vi "欧姆龙PLC通讯Fans UDP-写PLC寄存器编码-16bit寄存器.vi"(10 "数据U16":u16[](array[numeric]), 11 "起始地址16":string) -> (3 "写入数据编码":string)   [LabVIEW 2014]
panel:
  out "16bit寄存器个数":string
  out "字符串":string
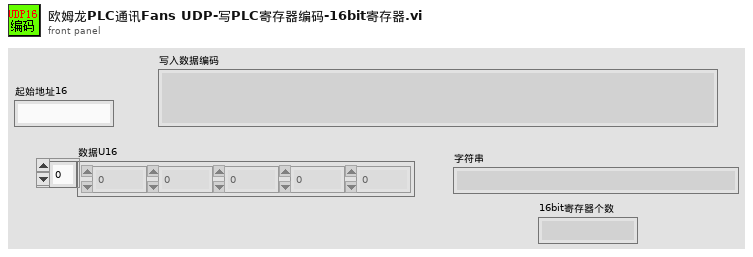
[diagram p1: front panel]
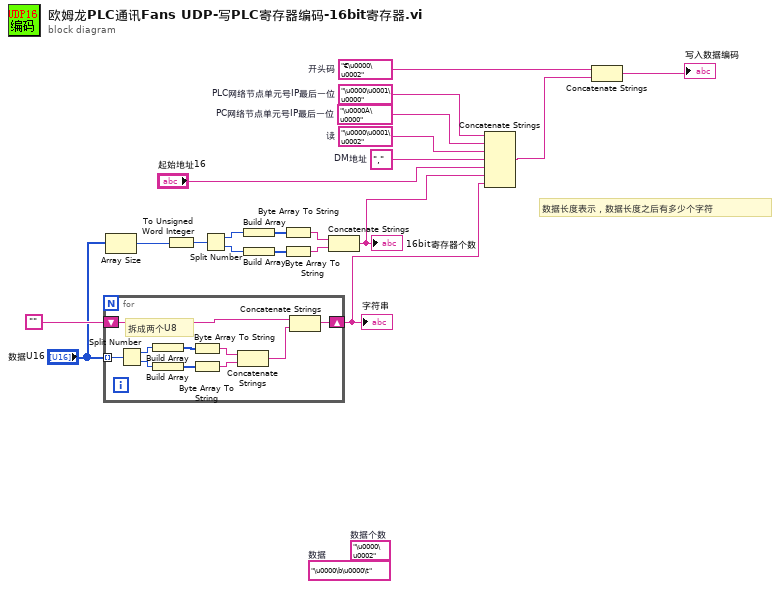
[diagram p0: block diagram]
diagram:
  w18 = "\u0000À\u0000"  # PC网络节点单元号IP最后一位
  w17 = "\u0000\u0001\u0000"  # PLC网络节点单元号IP最后一位
  w16 = "€\u0000\u0002"  # 开头码
  (unwired) "\u0000\b\u0000\t"  # 数据
  (unwired) "\u0000\u0002"  # 数据个数
  w14 = "‚"  # DM地址
  w13 = "\u0000\u0001\u0002"  # 读
  # "数据长度表示，数据长度之后有多少个字符"
  n1 = for {
    tunnel: "数据U16" -> [w21] mode=indexing
    shift-right: [w23] -> w1
    shift-left: "" -> [w24]
    # "拆成两个U8"
    n2 = Split Number(x=w21) -> (hi(x)=w30:u8, lo(x)=w29:u8)
    n3 = Build Array(w30) -> (w28:u8[])
    n4 = Build Array(w29) -> (w27:u8[])
    n5 = Byte Array To String(unsigned byte array=w28) -> (string=w26:string)
    n6 = Byte Array To String(unsigned byte array=w27) -> (string=w25:string)
    n7 = Concatenate Strings(w26, w25) -> (w22:string)
    n8 = Concatenate Strings(w24, w22) -> (w23:string)
  }
  "字符串" <- w1
  n9 = Array Size(array="数据U16") -> (size(s)=w3:i32)
  n10 = To Unsigned Word Integer(number=w3) -> (unsigned 16bit integer=w5:u16)
  n11 = Split Number(x=w5) -> (hi(x)=w6:u8, lo(x)=w7:u8)
  n12 = Build Array(w6) -> (w8:u8[])
  n13 = Build Array(w7) -> (w9:u8[])
  n14 = Byte Array To String(unsigned byte array=w8) -> (string=w10:string)
  n15 = Byte Array To String(unsigned byte array=w9) -> (string=w11:string)
  n16 = Concatenate Strings(w10, w11) -> (w2:string)
  "16bit寄存器个数" <- w2
  n17 = Concatenate Strings(w17, w18, w13, w14, "起始地址16", w2, w1) -> (w19:string)
  n18 = Concatenate Strings(w16, w19) -> (→"写入数据编码":string)
